vi "ChangeDriveTrainDeadband.vi"(10 "Eliminate Deadband":bool, 11 "Drivetrain in":T1) -> (3 "Drivetrain out":T1)   [LabVIEW 2017]
uses:
  <vilib>/Rock Robotics/WPI/RobotDrive/WPI_RobotDriveDevRef.ctl
  <vilib>/Rock Robotics/WPI/MotorControl/WPI_MotorControlDeviceRef.ctl
  <vilib>/Rock Robotics/WPI/MotorControl/WPI_MotorControlType.ctl
  <vilib>/Rock Robotics/SystemInterfaces/DIO/FPGA_DIOPWMChannel.ctl
  <vilib>/Rock Robotics/WPI/PWM/WPI_PWMDeadband.ctl
  <vilib>/Rock Robotics/SystemInterfaces/DIO/FPGA_DIOChannel.ctl
  <vilib>/Rock Robotics/WPI/PWM/WPI_PWMDeadband_ms.ctl
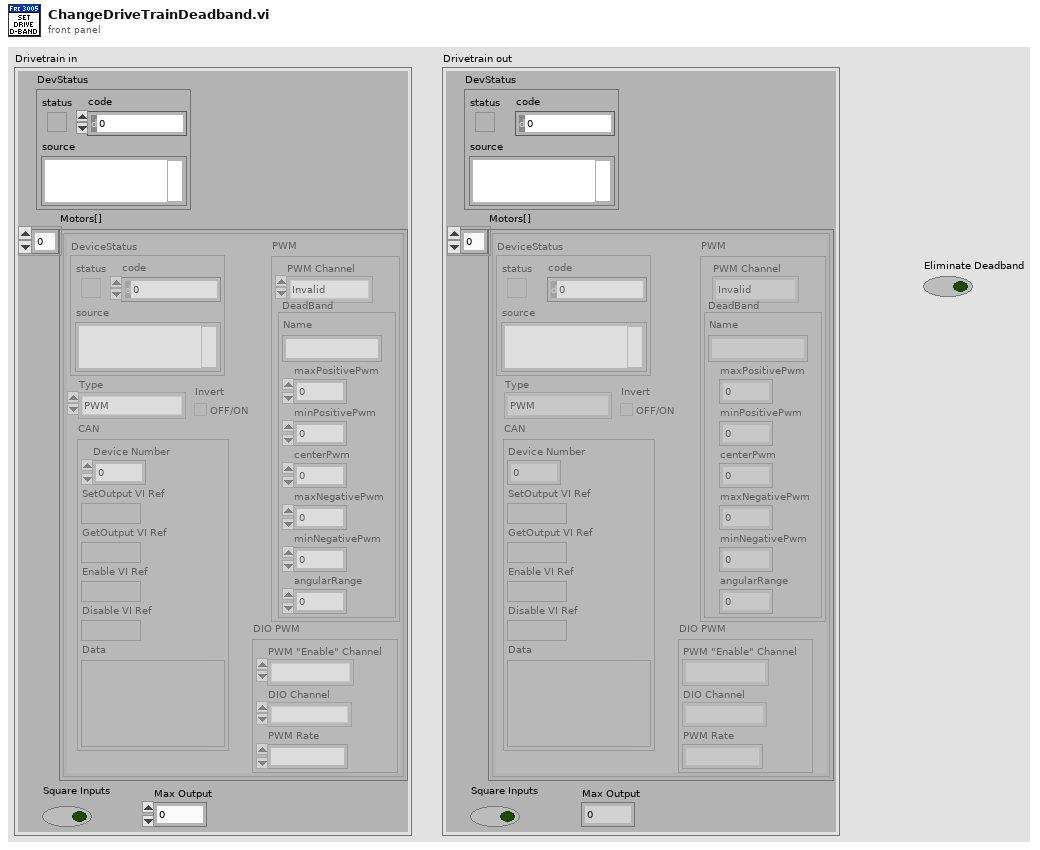
[diagram p1: front panel]
types:
  T1 = typedef "WPI_RobotDriveDevRef.ctl" = cluster{"DevStatus":errorcluster, "Motors[]":T2[], "Square Inputs":bool, "Max Output":dbl}
  T2 = typedef "WPI_MotorControlDeviceRef.ctl" = cluster{"DeviceStatus":errorcluster, "Type":T3, "PWM":cluster{"PWM Channel":T4, "DeadBand":T5}, "CAN":cluster{"Device Number":u8, "SetOutput VI Ref":variant, "GetOutput VI Ref":variant, "Enable VI Ref":variant, "Disable VI Ref":variant, "Data":variant}, "Invert":bool, "DIO PWM":cluster{"PWM \"Enable\" Channel":T4, "DIOChannel":T6, "PWM Rate":dbl}}
  T3 = typedef "WPI_MotorControlType.ctl" = enum16{"PWM", "CAN", "DIO PWM"}
  T4 = typedef "FPGA_DIOPWMChannel.ctl" = enum8{"PWM 0", "PWM 1", "PWM 2", "PWM 3", "PWM 4", "PWM 5", "PWM 6", "PWM 7", "PWM 8", "PWM 9", "PWM MXP 0", "PWM MXP 1", "PWM MXP 2", "PWM MXP 3", "PWM MXP 4", "PWM MXP 5", "PWM MXP 6", "PWM MXP 7", "PWM MXP 8", "PWM MXP 9", "Invalid"}
  T5 = typedef "WPI_PWMDeadband.ctl" = cluster{"Name":string, "maxPositivePwm":i32, "minPositivePwm":i32, "centerPwm":i32, "maxNegativePwm":i32, "minNegativePwm":i32, "angularRange":u16}
  T6 = typedef "FPGA_DIOChannel.ctl" = enum8{"DIO 0", "DIO 1", "DIO 2", "DIO 3", "DIO 4", "DIO 5", "DIO 6", "DIO 7", "DIO 8", "DIO 9", "DIO MXP 0", "DIO MXP 1", "DIO MXP 2", "DIO MXP 3", "DIO MXP 4", "DIO MXP 5", "DIO MXP 6", "DIO MXP 7", "DIO MXP 8", "DIO MXP 9", "DIO MXP 10", "DIO MXP 11", "DIO MXP 12", "DIO MXP 13", "DIO MXP 14", "DIO MXP 15", "SPI Port CS1", "SPI Port CS2", "SPI Port CS3", "SPI Port MISO", "SPI Port MOSI", "Invalid"}
  T7 = typedef "WPI_PWMDeadband_ms.ctl" = cluster{"Name":string, "maxPositivePwm":dbl, "minPositivePwm":dbl, "centerPwm":dbl, "maxNegativePwm":dbl, "minNegativePwm":dbl}
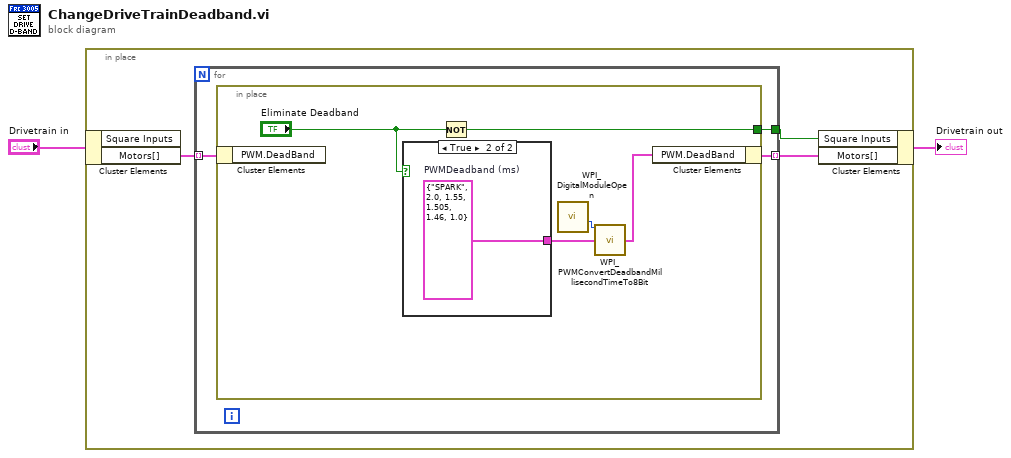
[diagram p0: block diagram]
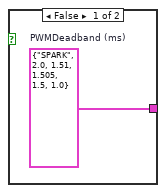
[diagram p2: hidden frame]
diagram:
  n1 = in-place {
    n2 = in-place-cluster #1("Drivetrain in") -> ("Motors[]"=w5:T2[])  [unwired: 1 out]
    n3 = for {
      tunnel: w5 -> [w8] mode=indexing
      tunnel: [w7] -> w4 mode=indexing
      tunnel: [w6] -> w3
      n4 = in-place {
        in-place-border: [w10] -> w6
        n5 = in-place-cluster #2(w8) -> ()  [unwired: 1 out]
        n6 = case shown="True" "Eliminate Deadband" {
          tunnel: [w14 w15] -> w13
          frame False {
            w14 = T7 {"Name"="SPARK", "maxPositivePwm"=2.0, "minPositivePwm"=1.51, "centerPwm"=1.505, "maxNegativePwm"=1.5, "minNegativePwm"=1.0}  # PWMDeadband (ms)
          }
          frame True {
            w15 = T7 {"Name"="SPARK", "maxPositivePwm"=2.0, "minPositivePwm"=1.55, "centerPwm"=1.505, "maxNegativePwm"=1.46, "minNegativePwm"=1.0}  # PWMDeadband (ms)
          }
        }
        n7 = Not(x="Eliminate Deadband") -> (.not. x?=w10:bool)
        n8 = call <vilib>:"WPI_DigitalModuleOpen.vi"() -> ("LoopTiming"=w11:u16)  [unwired: 2 in, 9 out]
        n9 = call <vilib>:"WPI_PWMConvertDeadbandMillisecondTimeTo8Bit.vi"("DIO Loop Timing (ticks)"=w11, "PWMDeadband (ms)"=w13) -> ("PWMDeadband Coefficient"=w12:T5)  [unwired: 13 in]
        n10 = in-place-cluster #2("PWM.DeadBand"=w12) -> (w7:T2)
      }
    }
    n11 = in-place-cluster #1("Square Inputs"=w3, "Motors[]"=w4) -> (→"Drivetrain out":T1)
  }
